vi "NumberMultiFile.vi"(1 "File number":i32, 2 "file name":string) -> (0 "Numbered File":string)   [LabVIEW 2022 SP3]
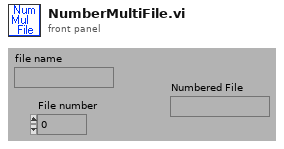
[diagram p1: front panel]
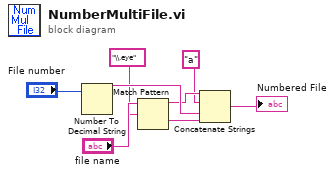
[diagram p0: block diagram]
diagram:
  n1 = Number To Decimal String(number="File number") -> (decimal integer string=w8:string)  [unwired: 1 out]
  n2 = Match Pattern(string="file name", regular expression="\\.eye") -> (before substring=w6:string, match substring=w7:string)  [unwired: 3 out]
  n3 = Concatenate Strings(w6, "a", w8, w7) -> (→"Numbered File":string)
